vi "direction.set.vi"(8 "error in (no error)":errorcluster, 9 "Direction SEQ":refnum<queue>, 11 "Game Board in":refnum<class "Game Board.lvclass">) -> (0 "error out":errorcluster, 3 "Game Board out":refnum<class "Game Board.lvclass">)   [LabVIEW 2020, in "Game Board.lvclass"]
uses:
  Game Board.lvclass
  Snake/Type Defs/Direction.ctl
  Game Board.lvclass/Game Board.ctl
  Snake/Snake.lvclass/Snake.ctl
  Snake/Snake.lvclass
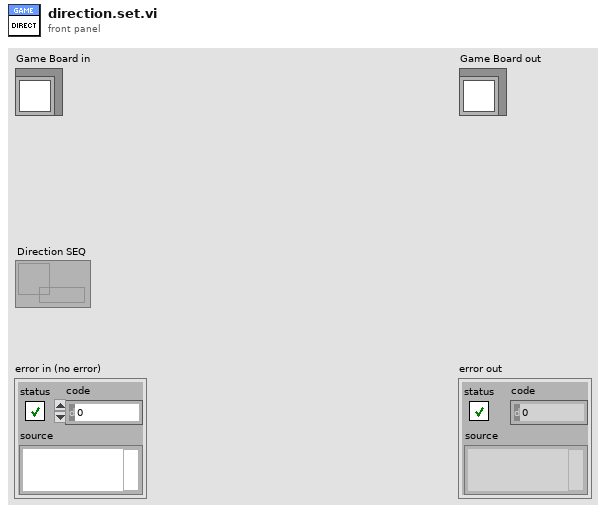
[diagram p1: front panel]
types:
  T1 = typedef "Direction.ctl" = enum16{"Up", "Down", "Left", "Right"}
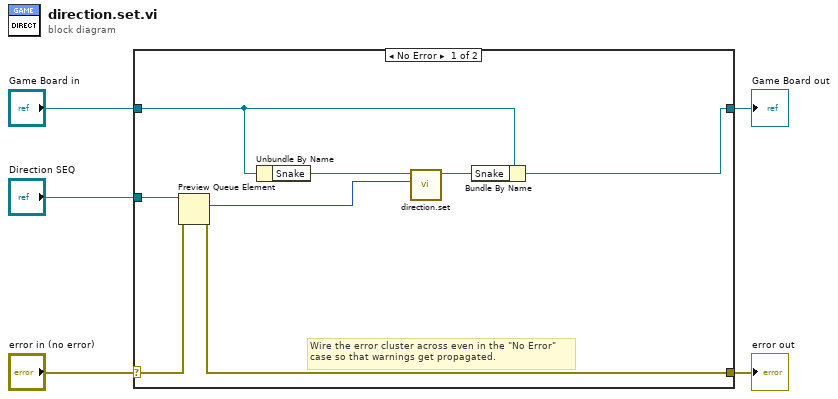
[diagram p0: block diagram]
diagram:
  n1 = case shown="No Error" "error in (no error)" {
    selector: "error in (no error)" -> [w7 w15]
    tunnel: [w6 w15] -> w4
    tunnel: [w10 w14] -> w2
    tunnel: "Game Board in" -> [w11 w14]
    tunnel: "Direction SEQ" -> [w13 _]
    frame No Error {
      # "Wire the error cluster across even in the \"No Error\"\ncase so that warnings get propagated."
      n2 = Preview Queue Element(queue=w13, error in (no error)=w7) -> (element=w8:T1, error out=w6:errorcluster)  [unwired: 1 in, 2 out]
      n3 = Unbundle By Name(w11) -> ("Snake"=w12:refnum<class "Snake.lvclass">)
      n4 = call "direction.set.vi"("Direction"=w8, "Snake in"=w12) -> ("Snake out"=w9:refnum<class "Snake.lvclass">)  [unwired: 8 in, 1 out]
      n5 = Bundle By Name(cluster=w11, "Snake"=w9) -> (w10:refnum<class "Game Board.lvclass">)
    }
    frame Error {
    }
  }
  "error out" <- w4
  "Game Board out" <- w2
